vi "Master_CalculateOffset.vi"(1 "Acceleration":dbl) -> (0 "Offset":dbl)   [LabVIEW 2018]
uses:
  <vilib>/Analysis/baseanly.llb/Mean (DBL).vi
  <vilib>/Analysis/NI_AALBase.lvlib
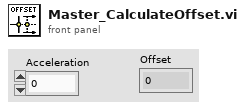
[diagram p1: front panel]
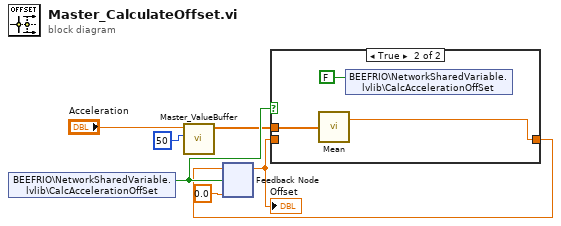
[diagram p0: block diagram]
diagram:
  n1 = shared-variable "BEEFRIO\\NetworkSharedVariable.lvlib\\CalcAccelerationOffSet"() -> (w4:bool)  [unwired: 1 in, 1 out]
  n2 = call "Master_ValueBuffer.vi"("n"=50, "new value"="Acceleration") -> ("Last n values"=w3:dbl[])  [unwired: 9 in]
  n3 = feedback #1(sgl 0.0 ("mean")) -> (w1:dbl)
  "Offset" <- w1
  n4 = case shown="True" w4 {
    tunnel: w3 -> [_ w10]
    tunnel: [w8 w9] -> w2
    tunnel: w1 -> [w8 _]
    frame False {
    }
    frame True {
      n5 = call-poly <vilib>:"Mean.vi"("X"=w10) -> ("mean"=w9:dbl)  [unwired: 1 out]
      n6 = shared-variable "BEEFRIO\\NetworkSharedVariable.lvlib\\CalcAccelerationOffSet"(FALSE ("CalcAccelerationOffset")) -> ()  [unwired: 1 in, 1 out]
    }
  }
  n7 = feedback-in #1(w2, w4) -> ()
